vi "List Baristas.vi"(8 "error in (no error)":errorcluster, 11 "Coffee Shop in":refnum<class "Coffee Shop.lvclass">) -> (0 "error out":errorcluster, 2 "Names":string[](array[string]), 3 "Coffee Shop out":refnum<class "Coffee Shop.lvclass">)   [LabVIEW 2020, in "Coffee Shop.lvclass"]
uses:
  Coffee Shop.lvclass
  Roles.ctl
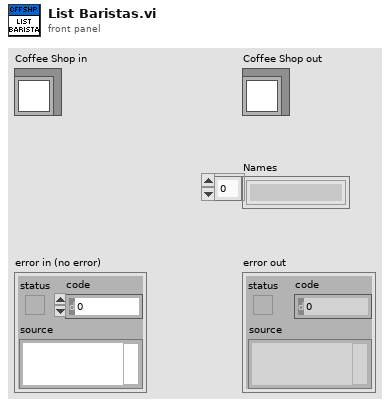
[diagram p1: front panel]
types:
  T1 = typedef "Coffee Shop.lvclass/Roles.ctl" = enum16{"Customer", "Barista", "Cashier"}
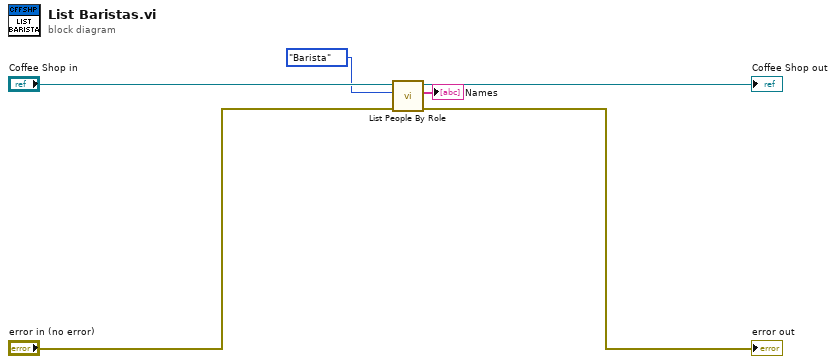
[diagram p0: block diagram]
diagram:
  n1 = call "List People By Role.vi"("error in (no error)"="error in (no error)", "Roles"=Roles."Barista", "Coffee Shop In"="Coffee Shop in") -> ("error out"=→"error out":errorcluster, "Names"=→"Names":string[], "Coffee Shop Out"=→"Coffee Shop out":refnum<class "Coffee Shop.lvclass">)  [unwired: 6 in]
